vi "scale.vi"(11 "Coords in":T1) -> (3 "Coords out":T1)   [LabVIEW 2021]
uses:
  <vilib>/Utility/miscctls.llb/LVPoint32TypeDef.ctl
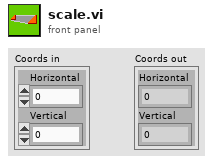
[diagram p1: front panel]
types:
  T1 = typedef "LVPoint32TypeDef.ctl" = cluster{"Horizontal":i32, "Vertical":i32}
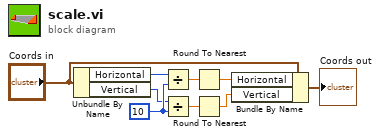
[diagram p0: block diagram]
diagram:
  w4 = 10 ("y")
  n1 = Unbundle By Name("Coords in") -> ("Horizontal"=w2:i32, "Vertical"=w3:i32)
  n2 = Divide(x=w2, y=w4) -> (x/y=w5:dbl)
  n3 = Divide(x=w3, y=w4) -> (x/y=w6:dbl)
  n4 = Round To Nearest(number=w5) -> (nearest integer value=w7:dbl)
  n5 = Round To Nearest(number=w6) -> (nearest integer value=w8:dbl)
  n6 = Bundle By Name(cluster="Coords in", "Horizontal"=w7, "Vertical"=w8) -> (→"Coords out":T1)
